vi "New Event.vi"(8 "error in (no error)":errorcluster, 9 "Is Repeat Attempt":bool, 10 "Event":T1, 11 "Controller in":refnum<class "Controller.lvclass">) -> (0 "error out":errorcluster, 3 "Controller out":refnum<class "Controller.lvclass">)   [LabVIEW 2019, in "Controller.lvlib" / "Controller.lvclass"]
uses:
  Controller.lvclass
  Sensors/Detector/Event.ctl
  Controller.lvclass/Controller.ctl
  Logger/Logger Messages/Log Event Msg/Log Event Msg.lvclass/Log Event Msg.ctl
  <vilib>/ActorFramework/Message Enqueuer/Message Enqueuer.lvclass/Message Enqueuer.ctl
  <vilib>/ActorFramework/Message Enqueuer/Enqueue.vi
  Logger/Logger Messages/Log Event Msg/Log Event Msg.lvclass
  C:/Program Files (x86)/National Instruments/LabVIEW 2019/vi.lib/ActorFramework/Message/Message.lvclass
  <vilib>/ActorFramework/Message Priority Queue/Priority Enqueue.vi
  Sensors/Detector/Muon Detector.lvclass
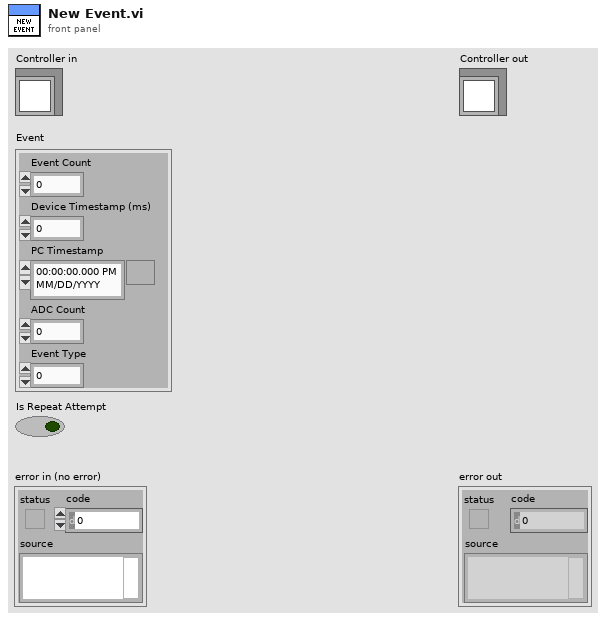
[diagram p1: front panel]
types:
  T1 = typedef "Muon Detector.lvclass/Event.ctl" = cluster{"Event Count":i32, "Device Timestamp (ms)":i32, "PC Timestamp":timestamp, "ADC Count":i32, "Event Type":u8}
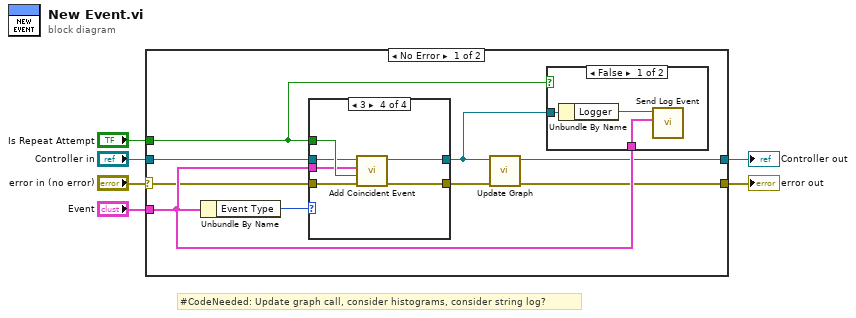
[diagram p0: block diagram]
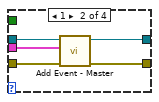
[diagram p4: hidden frame]
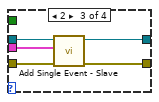
[diagram p5: hidden frame]
diagram:
  # "#CodeNeeded: Update graph call, consider histograms, consider string log?"
  n1 = case shown="No Error" "error in (no error)" {
    selector: "error in (no error)" -> [w12 w38]
    tunnel: [w10 w38] -> w5
    tunnel: [w9 w37] -> w3
    tunnel: "Controller in" -> [w13 w37]
    tunnel: "Event" -> [w15 _]
    tunnel: "Is Repeat Attempt" -> [w7 _]
    frame No Error {
      n2 = Unbundle By Name(w15) -> ("Event Type"=w14:u8)
      n3 = case shown="3" w14 {
        tunnel: w13 -> [w20 w25 w30 w34]
        tunnel: w15 -> [_ w24 w29 w35]
        tunnel: w12 -> [w19 w23 w28 w31]
        tunnel: [w19 w21 w27 w32] -> w11
        tunnel: [w20 w22 w26 w33] -> w8
        tunnel: w7 -> [_ _ _ w36]
        frame 0, Default {
          # "#Error: Can't get here"
        }
        frame 1 {
          n4 = call "Add Event - Master.vi"("error in (no error)"=w23, "Event"=w24, "Controller in"=w25) -> ("error out"=w21:errorcluster, "Controller out"=w22:refnum<class "Controller.lvclass">)  [unwired: 7 in]
        }
        frame 2 {
          n5 = call "Add Single Event - Slave.vi"("error in (no error)"=w28, "Event"=w29, "Controller in"=w30) -> ("error out"=w27:errorcluster, "Controller out"=w26:refnum<class "Controller.lvclass">)  [unwired: 7 in]
        }
        frame 3 {
          n6 = call "Add Coincident Event.vi"("error in (no error)"=w31, "Is Repeat Attempt"=w36, "Event"=w35, "Controller in"=w34) -> ("error out"=w32:errorcluster, "Controller out"=w33:refnum<class "Controller.lvclass">)  [unwired: 6 in]
        }
      }
      n7 = call "Update Graph.vi"("error in (no error)"=w11, "Controller in"=w8) -> ("error out"=w10:errorcluster, "Controller out"=w9:refnum<class "Controller.lvclass">)  [unwired: 8 in]
      n8 = case shown="False" w7 {
        tunnel: w15 -> [w18 _]
        tunnel: w8 -> [w17 _]
        frame False {
          n9 = Unbundle By Name(w17) -> ("Logger"=w16:refnum<class "Message Enqueuer.lvclass">)
          n10 = call "Send Log Event.vi"("Event"=w18, "Message Enqueuer"=w16) -> ()  [unwired: 8 in, 2 out]
        }
        frame True {
        }
      }
    }
    frame Error {
    }
  }
  "error out" <- w5
  "Controller out" <- w3
